vi "wave to DBL matrix.vi"(10 "data":waveform(dbl)[](array[waveform])) -> (2 "data array":dbl[][](array[numeric]))   [LabVIEW 2012]
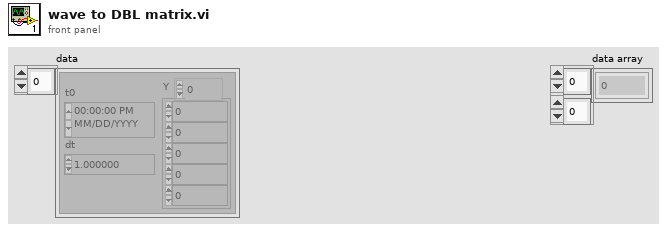
[diagram p1: front panel]
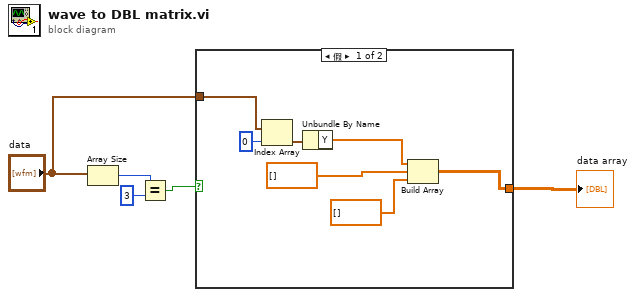
[diagram p0: block diagram]
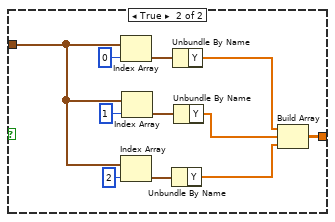
[diagram p2: hidden frame]
diagram:
  n1 = Array Size(array="data") -> (size(s)=w4:i32)
  n2 = Equal?(x=w4, y=3) -> (x = y?=w2:bool)
  n3 = case shown="假" w2 {
    tunnel: "data" -> [w11 w23]
    tunnel: [w8 w13] -> w1
    frame False {
      n4 = Index Array(array=w11, index=0 ("索引")) -> (element=w10:waveform(dbl))
      n5 = Unbundle By Name(w10) -> ("Y"=w9:dbl[])
      n6 = Build Array(w9, dbl[] [] ("元素"), dbl[] [] ("元素")) -> (w8:dbl[][])
    }
    frame True {
      n7 = Index Array(array=w23, index=0 ("索引")) -> (element=w19:waveform(dbl))
      n8 = Index Array(array=w23, index=2 ("索引")) -> (element=w17:waveform(dbl))
      n9 = Index Array(array=w23, index=1 ("索引")) -> (element=w18:waveform(dbl))
      n10 = Unbundle By Name(w17) -> ("Y"=w14:dbl[])
      n11 = Unbundle By Name(w19) -> ("Y"=w16:dbl[])
      n12 = Unbundle By Name(w18) -> ("Y"=w15:dbl[])
      n13 = Build Array(w16, w15, w14) -> (w13:dbl[][])
    }
  }
  "data array" <- w1
